vi "WriteInFileArchive.vi"(8 "error in (no error)":errorcluster, 10 "Строка таблицы":string[](array[string]), 11 "Archive in":refnum<class "Archive.lvclass">) -> (0 "error out":errorcluster, 3 "Archive out":refnum<class "Archive.lvclass">)   [LabVIEW 2010, in "Archive.lvclass"]
uses:
  Archive.lvclass
  Archive.lvclass/Archive.ctl
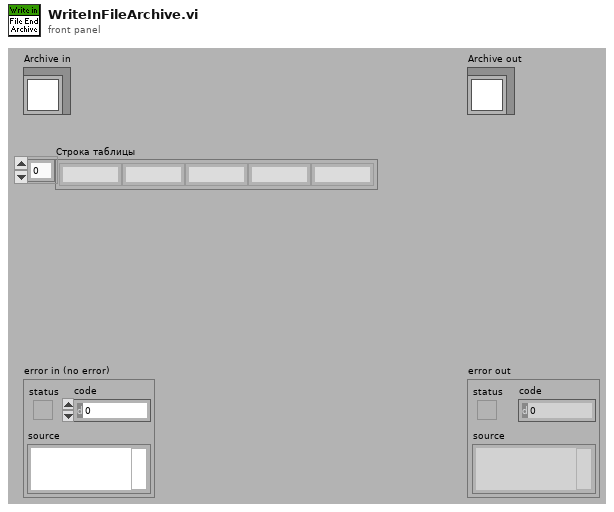
[diagram p1: front panel]
types:
  T1 = enum16{"big-endian, network order", "native, host order", "little-endian"}
  T2 = enum16{"open", "replace", "create", "open or create", "replace or create", "replace or create with confirmation"}
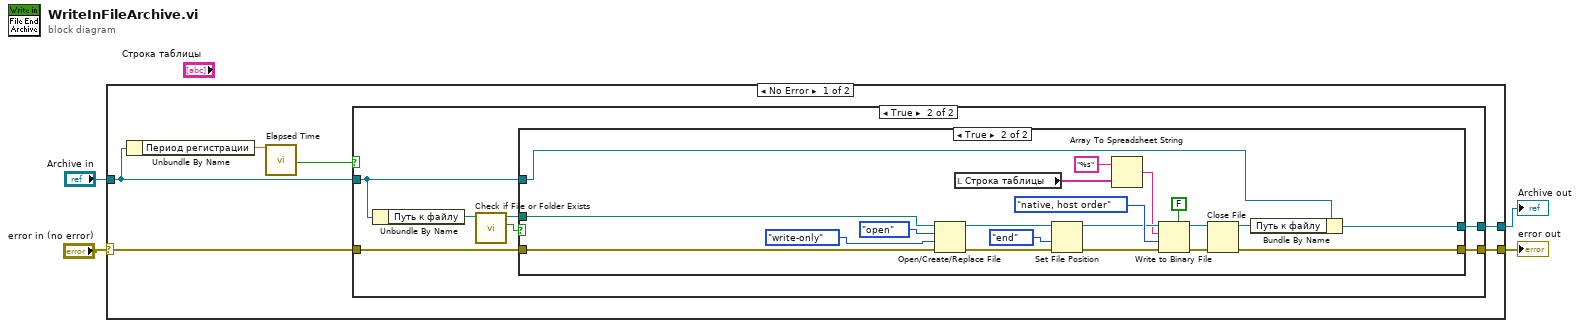
[diagram p0: block diagram]
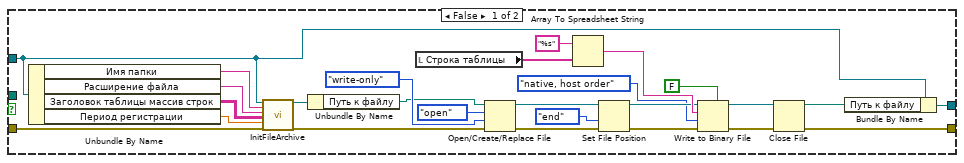
[diagram p3: hidden frame]
diagram:
  n1 = case shown="No Error" "error in (no error)" {
    selector: "error in (no error)" -> [w10 w67]
    tunnel: [w9 w67] -> w3
    tunnel: [w8 w66] -> w1
    tunnel: "Archive in" -> [w7 w66]
    frame No Error {
      n2 = Unbundle By Name(w7) -> ("Период регистрации"=w6:dbl)
      n3 = call "Elapsed Time"("Time Target (s)"=w6) -> ("Time has Elapsed"=w5:bool)  [unwired: 11 in, 7 out]
      n4 = case shown="True" w5 {
        tunnel: w10 -> [w11 w19]
        tunnel: [w11 w18] -> w9
        tunnel: [w12 w17] -> w8
        tunnel: w7 -> [w12 w13]
        frame False {
        }
        frame True {
          n5 = Unbundle By Name(w13) -> ("Путь к файлу"=w16:path)
          n6 = call <vilib>:"Check if File or Folder Exists.vi"("path"=w16) -> ("file or folder exists?"=w15:bool, "dup path"=w14:path)  [unwired: 8 in, 1 out]
          n7 = case shown="True" w15 {
            tunnel: w19 -> [w42 w55]
            tunnel: [w21 w53] -> w18
            tunnel: w13 -> [w26 w52]
            tunnel: [w25 w50] -> w17
            tunnel: w14 -> [_ w46]
            frame False {
              n8 = Unbundle By Name(w26) -> ("Имя папки"=w45:string, "Расширение файла"=w44:string, "Заголовок таблицы массив строк"=w43:string[][], "Период регистрации"=w20:dbl)
              n9 = call-dynamic "InitFileArchive.vi"("Archive In"=w26, "Имя папки"=w45, "Расширение имени файла"=w44, "Заголовок таблицы"=w43, "Период регистрации"=w20, "error in (no error)"=w42) -> ("Archive out"=w41:refnum<class "Archive.lvclass">, "error out"=w31:errorcluster)  [unwired: 12 in]
              n10 = Unbundle By Name(w41) -> ("Путь к файлу"=w36:path)
              n11 = local read "Строка таблицы"() -> (w40:string[])
              n12 = Open/Create/Replace File(file path (use dialog)=w36, error in=w31, operation (0:open)=T2."open", access (0:read/write)=enum16{"read/write", "read-only", "write-only"}."write-only") -> (refnum out=w33:refnum<file>, error out=w32:errorcluster)  [unwired: 2 in, 1 out]
              n13 = Array To Spreadsheet String(array=w40, 3:"%s") -> (spreadsheet string=w30:string)  [unwired: 1 in]
              n14 = Set File Position(refnum=w33, from (0:start)=enum16{"start", "end", "current"}."end", error in=w32) -> (refnum out=w29:refnum<file>, error out=w28:errorcluster)  [unwired: 1 in]
              n15 = Write to Binary File(file (use dialog)=w29, data=w30, error in=w28, 5:FALSE ("prepend array or string size? (T)"), 9:T1."native, host order" ("byte order (0:big-endian, network order)")) -> (refnum out=w24:refnum<file>, error out=w23:errorcluster)  [unwired: 1 in, 1 out]
              n16 = Close File(refnum=w24, error in=w23) -> (path=w22:path, error out=w21:errorcluster)
              n17 = Bundle By Name(cluster=w26, "Путь к файлу"=w22) -> (w25:refnum<class "Archive.lvclass">)
            }
            frame True {
              n18 = Open/Create/Replace File(file path (use dialog)=w46, error in=w55, operation (0:open)=T2."open", access (0:read/write)=enum16{"read/write", "read-only", "write-only"}."write-only") -> (refnum out=w58:refnum<file>, error out=w54:errorcluster)  [unwired: 2 in, 1 out]
              n19 = local read "Строка таблицы"() -> (w47:string[])
              n20 = Set File Position(refnum=w58, from (0:start)=enum16{"start", "end", "current"}."end", error in=w54) -> (refnum out=w60:refnum<file>, error out=w61:errorcluster)  [unwired: 1 in]
              n21 = Array To Spreadsheet String(array=w47, 3:"%s") -> (spreadsheet string=w48:string)  [unwired: 1 in]
              n22 = Write to Binary File(file (use dialog)=w60, data=w48, error in=w61, 5:FALSE ("prepend array or string size? (T)"), 9:T1."native, host order" ("byte order (0:big-endian, network order)")) -> (refnum out=w59:refnum<file>, error out=w64:errorcluster)  [unwired: 1 in, 1 out]
              n23 = Close File(refnum=w59, error in=w64) -> (path=w51:path, error out=w53:errorcluster)
              n24 = Bundle By Name(cluster=w52, "Путь к файлу"=w51) -> (w50:refnum<class "Archive.lvclass">)
            }
          }
        }
      }
    }
    frame Error {
    }
  }
  "error out" <- w3
  "Archive out" <- w1
